vi "Histogram Window.vi"() -> ()   [LabVIEW 2019, in "Histogram Window.lvlib"]
uses:
  Histogram Window.lvlib
  Histogram Window Q Element v2.ctl
  Histogram Window Q Action v2.ctl
  Fits/Fit Plot Request Information.ctl
  <vilib>/Utility/miscctls.llb/LVPointDoubleTypeDef.ctl
  Fits/Fit Models.ctl
  <vilib>/Utility/miscctls.llb/LVPoint32TypeDef.ctl
  ALiX/Updated Plot Info.ctl
  Graphs/Plot Style 3.ctl
  Plot Histogram.ctl
  Graphs/XY Graph/XY Graph Add-Ons.lvlib
  Notebook/Notebook.lvlib
  Rich Text Box/Rich Text Box.lvlib
  Graphs/Plot Editor/Plot Editor.lvlib
panel:
  out "Histogram Graph TipStrip":string caption="Histogram TipStrip"
  out "Histogram Graph":cluster{"Axis":dbl[], "Histogram":dbl[]}[](graph)
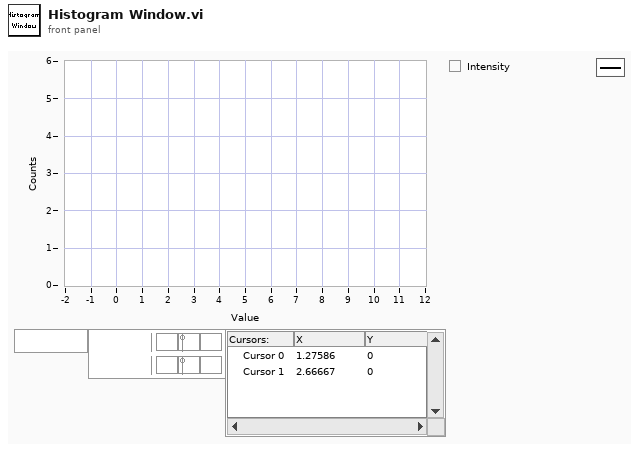
[diagram p1: front panel]
types:
  T1 = typedef "Histogram Window.lvlib/Histogram Window Q Element v2.ctl" = cluster{"Histogram Window Q Action":T2, "Data":variant}
  T2 = typedef "Histogram Window.lvlib/Histogram Window Q Action v2.ctl" = enum16{"Initialization", "Add Histogram", "Delete Histogram", "Delete Selected Histograms", "Clear Graph", "Change Bin Size", "Invert Histogram", "Update Graph", "Edit Plot", "Plot Fit", "Export XYGraph to Notebook", "Select All Plots", "Deselect All Plots", "Invert Plots Selection", "Set Style of Selected Plots", "Save Plot", "Save Selected Plots", "Save All Plots", "Quit"}
  T3 = cluster{"Event Registration Refnum":refnum<event-registration>}
  T4 = typedef "Histogram Window.lvlib/Updated Plot Info.ctl" = cluster{"Plot Index":i32, "Plot Name":string, "# Plots":i32, "Plot Style":T5}
  T5 = typedef "Plot Style 3.ctl" = cluster{"Plot Style":enum16{"unchanged", "Line", "Symbol", "Line + Symbol", "Histogram", "Histogram + Symbol"}, "Histogram Type":enum16{"unchanged", "Left Bound", "Center", "Right Bound"}, "Line Tickness":enum16{"unchanged", "Thin", "1 pixel", "2 pixel", "3 pixel", "4 pixel", "5 pixel"}, "Line Style":enum16{"unchanged", "Plain", "Long Dash", "Short Dash", "Long-Short Dash", "Long-Short-Short Dash"}, "Point Style":enum16{"unchanged", "None", "Empty Circle", "Filled Circle", "Thick Circle", "Dotted Circle", "Empty Square", "Filled Square", "Thick Square", "Dotted Square", "Small Filled Square", "Dot", "Cross", "Tiny Cross", "Large X", "Small x", "Diamond", "Small Empty Square"}, "Line Color":u32, "Point Color":u32, "Anti-aliased":bool, "Line Color Chooser":enum16{"unchanged", "Color Box", "Color List"}, "Point Color Chooser":enum16{"unchanged", "Color Box", "Color List"}, "Line Color List":string, "Point Color List":string}
  T6 = typedef "Histogram Window.lvlib/Plot Histogram.ctl" = cluster{"Plot Name":string, "Histogram":cluster{"Axis":dbl[], "Histogram":dbl[]}, "Plot Style":T5}
  T7 = typedef "LVPoint32TypeDef.ctl" = cluster{"Horizontal":i32, "Vertical":i32}
  T8 = typedef "Fit Plot Request Information.ctl" = cluster{"XY Graph Ref":refnum<vi>, "Mouse Coordinates":T9, "Fit Model":T10, "Plot Index":i32}
  T9 = typedef "LVPointDoubleTypeDef.ctl" = cluster{"X":dbl, "Y":dbl}
  T10 = typedef "Fit Models.ctl" = enum16{"Select a Fit Model...", "           Single Peak", "Gaussian", "Asymmetric Gaussian", "Lorentzian", "Asymmetric Lorentzian", "Gaussian/Lorentzian", "Lorentzian/Gaussian", "           Double Peak", "Two Gaussians", "Two Asymmetric Gaussians", "Two H-Connected Gaussians", "Two T-Connected Gaussians", "Two H-Connected Asymmetric Gaussians", "Two T-Connected Asymmetric Gaussians", "           Triple Peak", "Three Gaussians", "Three Asymmetric Gaussians", "              Decays", "1-Exponential", "IRF*PSED", "2-Exponentials", "               ACF", "2D Gaussian ACF", "2D Gaussian + Blinking ACF", "2D Gaussian + Flow ACF", "3D Gaussian ACF", "3D Gaussian + Blinking ACF", "             Multiplot", "2D Gaussian ACF & 2D Gaussian + Flow ACF"}
  T11 = cluster{"CtlRef":refnum<vi>, "Select All Plots":bool}
  T12 = typedef "XY Graph Add-Ons.lvlib/XY Graph Refnum.ctl" = refnum<vi>
  T13 = typedef "Rich Text Box.lvlib/Text Formatting.ctl" = cluster{"Font":string, "Text Color":T14, "Text Background Color":T14, "Text Style":enum16{"Regular", "Bold", "Italic", "Underline", "Strikeout"}, "Font Size (Points)":dbl, "Text Alignment":i32}
  T14 = typedef "Rich Text Box.lvlib/Text Colors.ctl" = enum16{"Unchanged", "Black", "Blue", "Gray", "Green", "Red", "White"}
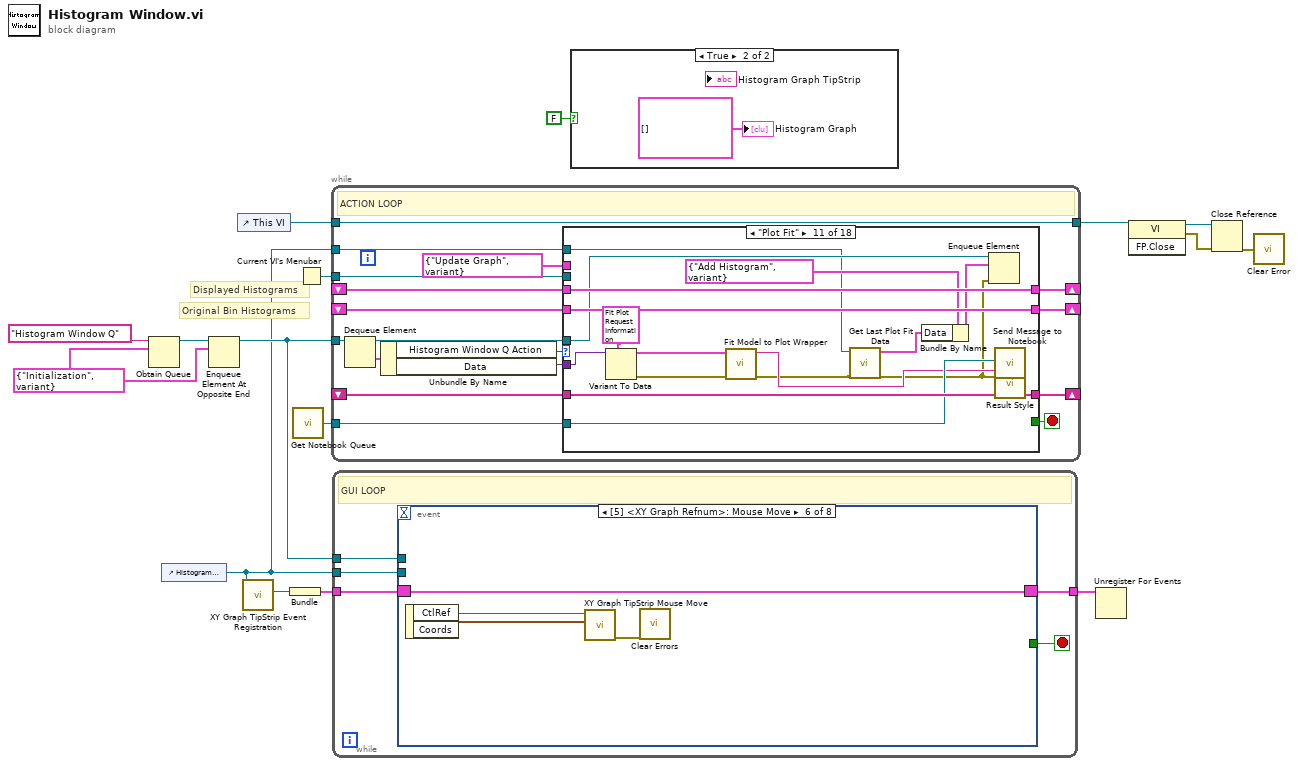
[diagram p0: block diagram]
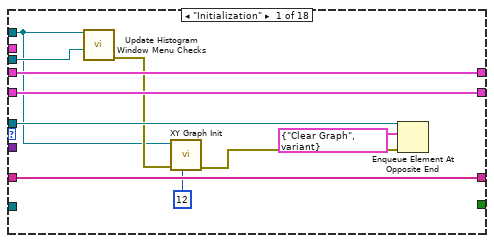
[diagram p3: hidden frame]
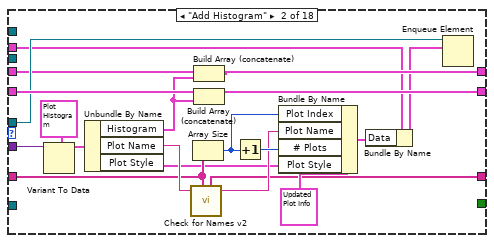
[diagram p4: hidden frame]
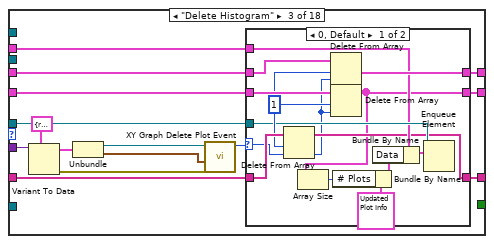
[diagram p5: hidden frame]
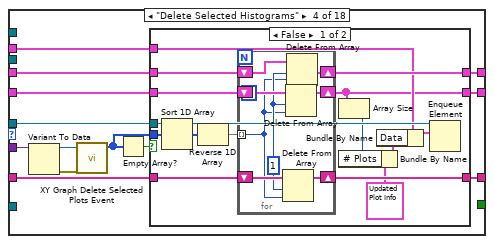
[diagram p7: hidden frame]
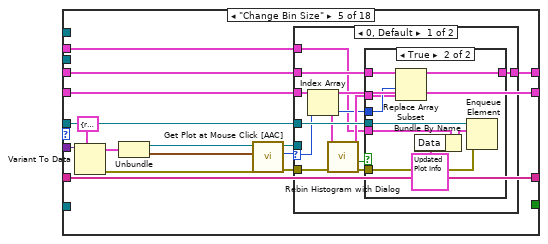
[diagram p9: hidden frame]
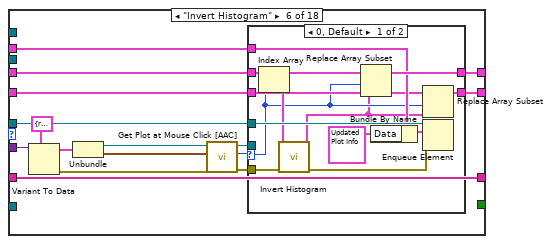
[diagram p12: hidden frame]
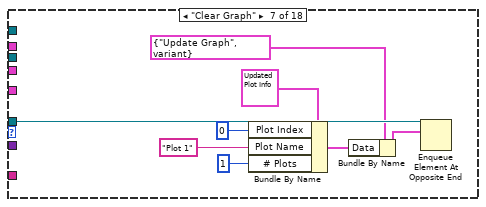
[diagram p14: hidden frame]
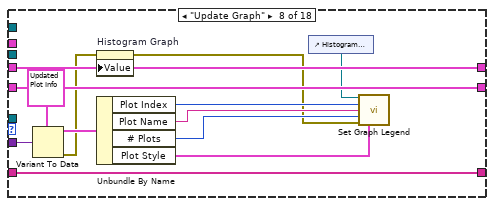
[diagram p15: hidden frame]
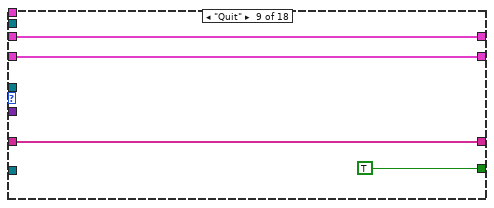
[diagram p16: hidden frame]
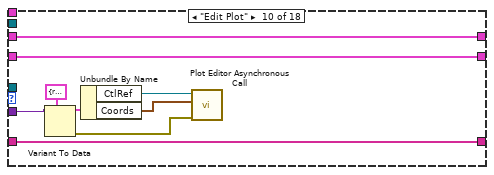
[diagram p17: hidden frame]
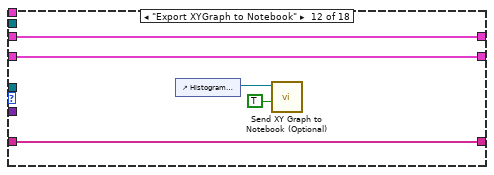
[diagram p18: hidden frame]
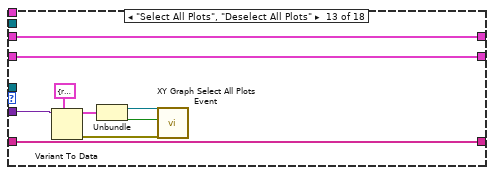
[diagram p19: hidden frame]
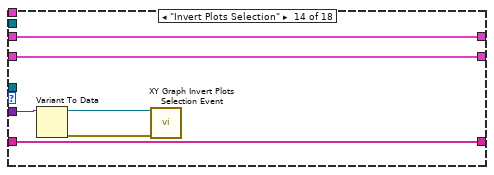
[diagram p20: hidden frame]
diagram:
  w11 = T1 {"Histogram Window Q Action"=enum."Initialization", "Data"=variant} ("ALEX TT Histogram Q Element")
  # "Displayed Histograms"
  # "Original Bin Histograms"
  n1 = Obtain Queue(name (unnamed)="Histogram Window Q", element data type=w11) -> (queue out=w15:refnum<queue>)  [unwired: 3 in, 2 out]
  n2 = control-ref of="Histogram Graph"() -> (w1:refnum<vi>)
  n3 = Enqueue Element At Opposite End(queue=w15, element=w11) -> (queue out=w12:refnum<queue>)  [unwired: 2 in, 2 out]
  n4 = control-ref of="This VI"() -> (w3:refnum<vi>)
  n5 = call "XY Graph TipStrip Event Registration.vi"("XY Graph Refnum"=w1) -> ("Event Registration Refnum"=w6:refnum<event-registration>)  [unwired: 8 in, 2 out]
  n6 = Bundle("Event Registration Refnum"=w6) -> (w9:T3)  [unwired: 1 in]
  n7 = call "Get Notebook Queue.vi"() -> ("Notebook Queue"=w10:refnum<queue>)  [unwired: 9 in]
  n8 = Current VI's Menubar() -> (w2:refnum<k9>)
  n9 = while {
    tunnel: w12 -> [w33]
    shift-right: [w27] -> _
    shift-left: _ -> [w28]
    shift-right: [w25] -> _
    shift-left: _ -> [w26]
    shift-right: [w22] -> _
    shift-left: _ -> [w23]
    tunnel: w10 -> [w20]
    tunnel: w3 -> [w19]
    tunnel: [w19] -> w7
    tunnel: w2 -> [w18]
    tunnel: w1 -> [w17]
    stop <- w30 stop-if-true
    # "ACTION LOOP"
    n10 = Dequeue Element(queue=w33) -> (queue out=w24:refnum<queue>, element=w32:T1)  [unwired: 2 in, 2 out]
    n11 = Unbundle By Name(w32) -> ("Histogram Window Q Action"=w31:T2, "Data"=w29:variant)
    n12 = case shown="\"Plot Fit\"" w31 {
      tunnel: [_ _ _ _ _ _ _ _ TRUE _ _ _ _ _ _ _ _ _] -> w30
      tunnel: w29 -> [_ w62 w78 w108 w149 w187 _ w220 _ w228 w253 _ w261 w270 w277 w296 w308 w319]
      tunnel: w28 -> [w40 w45 w71 w105 w144 w182 _ w223 w224 w236 w246 w256 w267 w273 w274 w303 w314 w325]
      tunnel: [w40 w46 w70 w104 w144 w182 _ w223 w224 w236 w246 w256 w267 w273 w274 w303 w314 w325] -> w27
      tunnel: w26 -> [w41 w63 w73 w107 w138 w173 _ w222 w225 w235 w251 w257 w266 w272 w282 w302 w313 w324]
      tunnel: [w41 w59 w72 w106 w138 w172 _ w222 w225 w235 w251 w257 w266 w272 w282 w302 w313 w324] -> w25
      tunnel: w24 -> [w43 w57 w68 w103 w139 w177 w210 _ _ _ w250 _ _ _ _ _ _ _]
      tunnel: w23 -> [w42 w56 w67 w102 w137 w176 _ w221 w226 w234 w252 w258 w265 w271 w281 w301 w312 w323]
      tunnel: [w42 w54 w66 w101 w136 w175 _ w221 w226 w234 w252 w258 w265 w271 w281 w301 w312 w323] -> w22
      tunnel: T1 {"Histogram Window Q Action"=enum."Update Graph", "Data"=variant} ("ALEX TT Histogram Q Element") -> [_ w50 w65 w100 w135 w174 _ _ _ _ _ _ _ _ _ _ _ _]
      tunnel: w20 -> [_ _ _ _ _ _ _ _ _ _ w244 _ _ _ _ w294 w306 w317]
      tunnel: w18 -> [w35 _ _ _ _ _ _ _ _ _ _ _ _ _ _ _ _ _]
      tunnel: w17 -> [w34 _ _ _ _ _ _ _ _ _ w239 _ _ _ _ _ _ _]
      frame "Initialization" {
        n13 = call "Update Histogram Window Menu Checks.vi"("menu reference"=w35, "XYGraph in"=w34) -> ("Error Out"=w36:errorcluster)  [unwired: 9 in]
        n14 = call "XY Graph Init.vi"("Max Legend Size (8)"=12 ("32bit integer"), "Error In"=w36, "XYGraph in"=w34) -> ("Error Out"=w38:errorcluster)  [unwired: 8 in]
        n15 = Enqueue Element At Opposite End(queue=w43, element=T1 {"Histogram Window Q Action"=enum."Clear Graph", "Data"=variant}, error in (no error)=w38) -> ()  [unwired: 1 in, 3 out]
      }
      frame "Add Histogram" {
        n16 = Variant To Data(type=T6 {"Plot Name"="", "Histogram"={"Axis"=[], "Histogram"=[]}, "Plot Style"={"Plot Style"=enum."Histogram + Symbol", "Histogram Type"=enum."Right Bound", "Line Tickness"=enum."unchanged", "Line Style"=enum."unchanged", "Point Style"=enum."unchanged", "Line Color"=0, "Point Color"=0, "Anti-aliased"=FALSE, "Line Color Chooser"=enum."unchanged", "Point Color Chooser"=enum."unchanged", "Line Color List"="", "Point Color List"=""}} ("output cluster"), Variant=w62) -> (data=w60:T6)  [unwired: 1 in, 1 out]
        n17 = Unbundle By Name(w60) -> ("Histogram"=w55:cluster{"Axis":dbl[], "Histogram":dbl[]}, "Plot Name"=w48:string, "Plot Style"=w44:T5)
        n18 = call "Check for Names v2.vi"("New Name"=w48, "Name List"=w45) -> ("New Name List"=w46:string[], "New Name"=w47:string)  [unwired: 4 in, 2 out]
        n19 = Array Size(array=w45) -> (size(s)=w53:i32)
        n20 = Build Array (concatenate)(w56, w55) -> (w54:cluster{"Axis":dbl[], "Histogram":dbl[]}[])
        n21 = Build Array (concatenate)(w63, w55) -> (w59:cluster{"Axis":dbl[], "Histogram":dbl[]}[])
        n22 = Increment(x=w53) -> (x+1=w58:i32)
        n23 = Bundle By Name(cluster=T4 {"Plot Index"=0, "Plot Name"="", "# Plots"=0, "Plot Style"={"Plot Style"=enum."Line + Symbol", "Histogram Type"=enum."Right Bound", "Line Tickness"=enum."Thin", "Line Style"=enum."unchanged", "Point Style"=enum."unchanged", "Line Color"=0, "Point Color"=0, "Anti-aliased"=FALSE, "Line Color Chooser"=enum."unchanged", "Point Color Chooser"=enum."unchanged", "Line Color List"="", "Point Color List"=""}} ("output cluster"), "Plot Index"=w53, "Plot Name"=w47, "# Plots"=w58, "Plot Style"=w44) -> (w51:T4)
        n24 = Bundle By Name(cluster=w50, "Data"=w51) -> (w52:T1)
        n25 = Enqueue Element(queue=w57, element=w52) -> ()  [unwired: 2 in, 3 out]
      }
      frame "Delete Histogram" {
        n26 = Variant To Data(type=cluster{"CtlRef":refnum<vi>, "Coords":T7} {"CtlRef"=refnum, "Coords"={"Horizontal"=0, "Vertical"=0}} ("output cluster"), Variant=w78) -> (data=w77:cluster{"CtlRef":refnum<vi>, "Coords":T7}, error out=w69:errorcluster)  [unwired: 1 in]
        n27 = Unbundle(w77) -> ("CtlRef"=w75:refnum<vi>, "Coords"=w74:T7)
        n28 = call "XY Graph Delete Plot Event.vi"("Error In"=w69, "Mouse Click Coordinates"=w74, "XYGraph Ref"=w75) -> ("Deleted Plot Index"=w64:i32)  [unwired: 4 in, 4 out]
        n29 = case shown="0, Default" w64 {
          selector: w64 -> [w81 _]
          tunnel: w73 -> [w92 w95]
          tunnel: [w79 w95] -> w72
          tunnel: w71 -> [w91 w94]
          tunnel: [w84 w94] -> w70
          tunnel: w68 -> [w87 _]
          tunnel: w67 -> [w90 w93]
          tunnel: [w89 w93] -> w66
          tunnel: w65 -> [w85 _]
          frame 0, Default {
            w88 = 1 ("length")
            n30 = Delete From Array(array=w91, length=w88, index=w81) -> (array with subset deleted=w84:string[])  [unwired: 1 out]
            n31 = Delete From Array(array=w90, length=w88, index=w81) -> (array with subset deleted=w89:cluster{"Axis":dbl[], "Histogram":dbl[]}[])  [unwired: 1 out]
            n32 = Delete From Array(array=w92, length=w88, index=w81) -> (array with subset deleted=w79:cluster{"Axis":dbl[], "Histogram":dbl[]}[])  [unwired: 1 out]
            n33 = Array Size(array=w79) -> (size(s)=w80:i32)
            n34 = Bundle By Name(cluster=T4 {"Plot Index"=-1, "Plot Name"="", "# Plots"=0, "Plot Style"={"Plot Style"=enum."Histogram + Symbol", "Histogram Type"=enum."Right Bound", "Line Tickness"=enum."unchanged", "Line Style"=enum."unchanged", "Point Style"=enum."unchanged", "Line Color"=0, "Point Color"=0, "Anti-aliased"=FALSE, "Line Color Chooser"=enum."unchanged", "Point Color Chooser"=enum."unchanged", "Line Color List"="", "Point Color List"=""}} ("output cluster"), "# Plots"=w80) -> (w83:T4)
            n35 = Bundle By Name(cluster=w85, "Data"=w83) -> (w86:T1)
            n36 = Enqueue Element(queue=w87, element=w86) -> ()  [unwired: 2 in, 3 out]
          }
          frame -1 {
          }
        }
      }
      frame "Delete Selected Histograms" {
        n37 = Variant To Data(Variant=w108) -> (data=w98:T12, error out=w99:errorcluster)  [unwired: 2 in]
        n38 = call "XY Graph Delete Selected Plots Event.vi"("Error In"=w99, "XYGraph Ref"=w98) -> ("Deleted Plot Indices"=w96:i32[])  [unwired: 5 in, 4 out]
        n39 = Empty Array?(array=w96) -> (empty?=w97:bool)
        n40 = case shown="False" w97 {
          tunnel: w107 -> [w123 w134]
          tunnel: [w112 w134] -> w106
          tunnel: w105 -> [w122 w133]
          tunnel: [w116 w133] -> w104
          tunnel: w103 -> [w119 _]
          tunnel: w102 -> [w121 w132]
          tunnel: [w120 w132] -> w101
          tunnel: w100 -> [w117 _]
          tunnel: w96 -> [w111 _]
          frame False {
            n41 = Sort 1D Array(array=w111) -> (sorted array=w110:i32[])
            n42 = Reverse 1D Array(array=w110) -> (reversed array=w109:i32[])
            n43 = for {
              shift-right: [w128] -> w120
              shift-left: w121 -> [w129]
              shift-right: [w125] -> w112
              shift-left: w123 -> [w131]
              shift-right: [w126] -> w116
              shift-left: w122 -> [w130]
              tunnel: w109 -> [w124] mode=indexing
              w127 = 1 ("length")
              n44 = Delete From Array(array=w130, length=w127, index=w124) -> (array with subset deleted=w126:string[])  [unwired: 1 out]
              n45 = Delete From Array(array=w131, length=w127, index=w124) -> (array with subset deleted=w125:cluster{"Axis":dbl[], "Histogram":dbl[]}[])  [unwired: 1 out]
              n46 = Delete From Array(array=w129, length=w127, index=w124) -> (array with subset deleted=w128:cluster{"Axis":dbl[], "Histogram":dbl[]}[])  [unwired: 1 out]
            }
            n47 = Array Size(array=w112) -> (size(s)=w113:i32)
            n48 = Bundle By Name(cluster=T4 {"Plot Index"=-1, "Plot Name"="", "# Plots"=0, "Plot Style"={"Plot Style"=enum."Histogram + Symbol", "Histogram Type"=enum."Right Bound", "Line Tickness"=enum."unchanged", "Line Style"=enum."unchanged", "Point Style"=enum."unchanged", "Line Color"=0, "Point Color"=0, "Anti-aliased"=FALSE, "Line Color Chooser"=enum."unchanged", "Point Color Chooser"=enum."unchanged", "Line Color List"="", "Point Color List"=""}} ("output cluster"), "# Plots"=w113) -> (w115:T4)
            n49 = Bundle By Name(cluster=w117, "Data"=w115) -> (w118:T1)
            n50 = Enqueue Element(queue=w119, element=w118) -> ()  [unwired: 2 in, 3 out]
          }
          frame True {
          }
        }
      }
      frame "Change Bin Size" {
        n51 = Variant To Data(type=cluster{"CtlRef":refnum<vi>, "Coords":T7} {"CtlRef"=refnum, "Coords"={"Horizontal"=0, "Vertical"=0}} ("output cluster"), Variant=w149) -> (data=w148:cluster{"CtlRef":refnum<vi>, "Coords":T7}, error out=w143:errorcluster)  [unwired: 1 in]
        n52 = Unbundle(w148) -> ("CtlRef"=w146:refnum<vi>, "Coords"=w145:T7)
        n53 = call "Get Plot at Mouse Click [AAC].vi"("error in (no error)"=w143, "Mouse Click Coordinates"=w145, "XYGraph Ref"=w146) -> ("error out"=w141:errorcluster, "Plot at Coordinates"=w142:i32, "XYGraph Ref"=w140:T12)  [unwired: 2 in, 4 out]
        n54 = case shown="0, Default" w142 {
          selector: w142 -> [w151 _]
          tunnel: w141 -> [w160 _]
          tunnel: w140 -> [_ _]
          tunnel: w139 -> [w159 _]
          tunnel: w138 -> [w157 _]
          tunnel: w137 -> [w154 w171]
          tunnel: [w153 w171] -> w136
          tunnel: w135 -> [w150 _]
          frame 0, Default {
            n55 = Index Array(array=w157, index=w151) -> (element=w156:cluster{"Axis":dbl[], "Histogram":dbl[]})
            n56 = call "Rebin Histogram with Dialog.vi"("error in (no error)"=w160, "Original Bin Histogram"=w156) -> ("error out"=w158:errorcluster, "OK?"=w155:bool, "Rebinned Histogram"=w152:cluster{"Axis":dbl[], "Histogram":dbl[]})  [unwired: 7 in]
            n57 = case shown="True" w155 {
              tunnel: w159 -> [_ w170]
              tunnel: w158 -> [_ w169]
              tunnel: w154 -> [w161 w168]
              tunnel: [w161 w167] -> w153
              tunnel: w152 -> [_ w165]
              tunnel: w151 -> [_ w166]
              tunnel: w150 -> [_ w164]
              frame False {
              }
              frame True {
                n58 = Replace Array Subset(array=w168, new element=w165, index=w166) -> (w167:cluster{"Axis":dbl[], "Histogram":dbl[]}[])
                n59 = Bundle By Name(cluster=w164, "Data"=T4 {"Plot Index"=-1, "Plot Name"="", "# Plots"=0, "Plot Style"={"Plot Style"=enum."Histogram + Symbol", "Histogram Type"=enum."Right Bound", "Line Tickness"=enum."unchanged", "Line Style"=enum."unchanged", "Point Style"=enum."unchanged", "Line Color"=0, "Point Color"=0, "Anti-aliased"=FALSE, "Line Color Chooser"=enum."unchanged", "Point Color Chooser"=enum."unchanged", "Line Color List"="", "Point Color List"=""}} ("Updated Plot Info")) -> (w163:T1)
                n60 = Enqueue Element(queue=w170, element=w163, error in (no error)=w169) -> ()  [unwired: 1 in, 3 out]
              }
            }
          }
          frame -1 {
          }
        }
      }
      frame "Invert Histogram" {
        n61 = Variant To Data(type=cluster{"CtlRef":refnum<vi>, "Coords":T7} {"CtlRef"=refnum, "Coords"={"Horizontal"=0, "Vertical"=0}} ("output cluster"), Variant=w187) -> (data=w186:cluster{"CtlRef":refnum<vi>, "Coords":T7}, error out=w181:errorcluster)  [unwired: 1 in]
        n62 = Unbundle(w186) -> ("CtlRef"=w184:refnum<vi>, "Coords"=w183:T7)
        n63 = call "Get Plot at Mouse Click [AAC].vi"("error in (no error)"=w181, "Mouse Click Coordinates"=w183, "XYGraph Ref"=w184) -> ("error out"=w179:errorcluster, "Plot at Coordinates"=w180:i32, "XYGraph Ref"=w178:T12)  [unwired: 2 in, 4 out]
        n64 = case shown="0, Default" w180 {
          selector: w180 -> [w190 _]
          tunnel: w179 -> [w200 _]
          tunnel: w178 -> [_ _]
          tunnel: w177 -> [w199 _]
          tunnel: w176 -> [w195 w202]
          tunnel: [w197 w202] -> w175
          tunnel: w174 -> [w196 _]
          tunnel: w173 -> [w191 w201]
          tunnel: [w188 w201] -> w172
          frame 0, Default {
            n65 = Index Array(array=w195, index=w190) -> (element=w194:cluster{"Axis":dbl[], "Histogram":dbl[]})
            n66 = call "Invert Histogram.vi"("error in (no error)"=w200, "Histogram"=w194) -> ("error out"=w198:errorcluster, "Inverted Histogram"=w189:cluster{"Axis":dbl[], "Histogram":dbl[]})  [unwired: 8 in]
            n67 = Replace Array Subset(array=w195, new element=w189, index=w190) -> (w197:cluster{"Axis":dbl[], "Histogram":dbl[]}[])
            n68 = Bundle By Name(cluster=w196, "Data"=T4 {"Plot Index"=-1, "Plot Name"="", "# Plots"=0, "Plot Style"={"Plot Style"=enum."Histogram + Symbol", "Histogram Type"=enum."Right Bound", "Line Tickness"=enum."unchanged", "Line Style"=enum."unchanged", "Point Style"=enum."unchanged", "Line Color"=0, "Point Color"=0, "Anti-aliased"=FALSE, "Line Color Chooser"=enum."unchanged", "Point Color Chooser"=enum."unchanged", "Line Color List"="", "Point Color List"=""}} ("output cluster")) -> (w193:T1)
            n69 = Replace Array Subset(array=w191, new element=w189, index=w190) -> (w188:cluster{"Axis":dbl[], "Histogram":dbl[]}[])
            n70 = Enqueue Element(queue=w199, element=w193, error in (no error)=w198) -> ()  [unwired: 1 in, 3 out]
          }
          frame -1 {
          }
        }
      }
      frame "Clear Graph" {
        n71 = Bundle By Name(cluster=T4 {"Plot Index"=0, "Plot Name"="", "# Plots"=0, "Plot Style"={"Plot Style"=enum."Histogram + Symbol", "Histogram Type"=enum."Right Bound", "Line Tickness"=enum."unchanged", "Line Style"=enum."unchanged", "Point Style"=enum."unchanged", "Line Color"=0, "Point Color"=0, "Anti-aliased"=FALSE, "Line Color Chooser"=enum."unchanged", "Point Color Chooser"=enum."unchanged", "Line Color List"="", "Point Color List"=""}} ("output cluster"), "Plot Index"=0, "Plot Name"="Plot 1", "# Plots"=1 ("# Legend Rows")) -> (w206:T4)
        n72 = Bundle By Name(cluster=T1 {"Histogram Window Q Action"=enum."Update Graph", "Data"=variant} ("ALEX TT Histogram Q Element"), "Data"=w206) -> (w208:T1)
        n73 = Enqueue Element At Opposite End(queue=w210, element=w208) -> ()  [unwired: 2 in, 3 out]
      }
      frame "Update Graph" {
        n74 = Variant To Data(type=T4 {"Plot Index"=0, "Plot Name"="", "# Plots"=0, "Plot Style"={"Plot Style"=enum."Histogram + Symbol", "Histogram Type"=enum."Right Bound", "Line Tickness"=enum."unchanged", "Line Style"=enum."unchanged", "Point Style"=enum."unchanged", "Line Color"=0, "Point Color"=0, "Anti-aliased"=FALSE, "Line Color Chooser"=enum."unchanged", "Point Color Chooser"=enum."unchanged", "Line Color List"="", "Point Color List"=""}} ("output cluster"), Variant=w220) -> (data=w218:T4, error out=w213:errorcluster)  [unwired: 1 in]
        n75 = property on="Histogram Graph" class="XYGraph (strict)"(error in=w213, "Value"=w221) -> (error out=w212:errorcluster)  [unwired: 1 in, 1 out]
        n76 = Unbundle By Name(w218) -> ("Plot Index"=w217:i32, "Plot Name"=w215:string, "# Plots"=w216:i32, "Plot Style"=w211:T5)
        n77 = control-ref of="Histogram Graph"() -> (w214:refnum<vi>)
        n78 = call "Set Graph Legend.vi"("XYGraph in"=w214, "Active Plot"=w217, "Plot Name"=w215, "# Plots"=w216, "error in (no error)"=w212, "Plot Style"=w211) -> ()  [unwired: 9 in, 1 out]
      }
      frame "Quit" {
      }
      frame "Edit Plot" {
        n79 = Variant To Data(type=cluster{"CtlRef":refnum<vi>, "Coords":T7} {"CtlRef"=refnum, "Coords"={"Horizontal"=0, "Vertical"=0}} ("output cluster"), Variant=w228) -> (data=w230:cluster{"CtlRef":refnum<vi>, "Coords":T7}, error out=w232:errorcluster)  [unwired: 1 in]
        n80 = Unbundle By Name(w230) -> ("CtlRef"=w233:refnum<vi>, "Coords"=w231:T7)
        n81 = call "Plot Editor Asynchronous Call.vi"("error in (no error)"=w232, "Coords"=w231, "XYGraph in"=w233) -> ()  [unwired: 5 in, 4 out]
      }
      frame "Plot Fit" {
        n82 = Variant To Data(type=T8 {"XY Graph Ref"=refnum, "Mouse Coordinates"={"X"=0.0, "Y"=0.0}, "Fit Model"=enum."Select a Fit Model...", "Plot Index"=-1} ("output cluster"), Variant=w253) -> (data=w242:T8, error out=w240:errorcluster)  [unwired: 1 in]
        n83 = call "Fit Model to Plot Wrapper.vi"("error in (no error)"=w240, "Fit Plot Info"=w242) -> ("error out"=w238:errorcluster, "Fit Result String"=w243:string)  [unwired: 8 in]
        n84 = call "Get Last Plot Fit Data.vi"("error in (no error)"=w238, "XYGraph in"=w239) -> ("error out"=w237:errorcluster, "Last Fit Data"=w247:T6)  [unwired: 8 in]
        n85 = Bundle By Name(cluster=T1 {"Histogram Window Q Action"=enum."Add Histogram", "Data"=variant} ("element"), "Data"=w247) -> (w248:T1)
        n86 = Enqueue Element(queue=w250, element=w248, error in (no error)=w237) -> ()  [unwired: 1 in, 3 out]
        n87 = call "Result Style.vi"() -> ("Default Text Formatting"=w241:T13)
        n88 = call "Send Message to Notebook.vi"("Notebook Queue"=w244, "Message"=w243, "Error In"=w237, "Text Formatting"=w241) -> ()  [unwired: 15 in, 1 out]
      }
      frame "Export XYGraph to Notebook" {
        n89 = control-ref of="Histogram Graph"() -> (w255:refnum<vi>)
        n90 = call "Send XY Graph to Notebook (Optional).vi"("Send Graph to Notebook?"=TRUE, "XYGraph in"=w255) -> ()  [unwired: 9 in, 1 out]
      }
      frame "Select All Plots", "Deselect All Plots" {
        n91 = Variant To Data(type=T11 {"CtlRef"=refnum, "Select All Plots"=TRUE} ("output cluster"), Variant=w261) -> (data=w264:T11, error out=w259:errorcluster)  [unwired: 1 in]
        n92 = Unbundle(w264) -> ("CtlRef"=w263:refnum<vi>, "Select All Plots"=w262:bool)
        n93 = call "XY Graph Select All Plots Event.vi"("Error In"=w259, "Select (T)/Deselect"=w262, "XYGraph Ref"=w263) -> ()  [unwired: 5 in, 4 out]
      }
      frame "Invert Plots Selection" {
        n94 = Variant To Data(Variant=w270) -> (data=w269:T12, error out=w268:errorcluster)  [unwired: 2 in]
        n95 = call "XY Graph Invert Plots Selection Event.vi"("Error In"=w268, "XYGraph Ref"=w269) -> ()  [unwired: 6 in, 4 out]
      }
      frame "Set Style of Selected Plots" {
        n96 = Variant To Data(type=refnum<vi> refnum ("XYGraph Ref"), Variant=w277) -> (data=w275:refnum<vi>)  [unwired: 1 in, 1 out]
        n97 = call "Plot Style Chooser Dialog.vi"() -> ("Plot Style out"=w280:T5, "Cancelled?"=w279:bool, "Error Out"=w278:errorcluster)  [unwired: 7 in]
        n98 = case shown="True" w279 {
          tunnel: w275 -> [_ w285]
          tunnel: w280 -> [_ w284]
          tunnel: w278 -> [_ w283]
          frame False {
          }
          frame True {
            n99 = call "XY Graph Set Style of Selected Plots.vi"("Error In"=w283, "Plot Style"=w284, "XYGraph Ref"=w285) -> ()  [unwired: 5 in, 4 out]
          }
        }
      }
      frame "Save Plot" {
        n100 = Variant To Data(type=cluster{"CtlRef":refnum<vi>, "Coords":T7} {"CtlRef"=refnum, "Coords"={"Horizontal"=0, "Vertical"=0}} ("output cluster"), Variant=w296) -> (data=w299:cluster{"CtlRef":refnum<vi>, "Coords":T7}, error out=w295:errorcluster)  [unwired: 1 in]
        n101 = Unbundle By Name(w299) -> ("CtlRef"=w297:refnum<vi>, "Coords"=w298:T7)
        n102 = call "XY Graph Save Plot Event.vi"("Error In"=w295, "Mouse Click Coordinates"=w298, "XYGraph Ref"=w297) -> ("Error Out"=w289:errorcluster, "Message"=w292:string, "File Path"=w286:path, "Plot Name"=w287:string)  [unwired: 3 in, 2 out]
        n103 = Format Into String(format string=" from %s saved as %s", initial string=w292, error in=w289, w287, w286) -> (resulting string=w290:string, error out=w288:errorcluster)
        n104 = call "Message Style.vi"() -> ("Message Formatting"=w293:T13)
        n105 = call "Send Message to Notebook.vi"("Notebook Queue"=w294, "Message"=w290, "Error In"=w288, "Text Formatting"=w293) -> ()  [unwired: 15 in, 1 out]
      }
      frame "Save Selected Plots" {
        n106 = Variant To Data(Variant=w308) -> (data=w311:T12, error out=w309:errorcluster)  [unwired: 2 in]
        n107 = call "XY Graph Save Selected Plots Event.vi"("Error In"=w309, "Save All Plots? (T)"=FALSE, "XYGraph Ref"=w311) -> ("Error Out"=w305:errorcluster, "Message"=w304:string)  [unwired: 3 in, 4 out]
        n108 = call "Message Style.vi"() -> ("Message Formatting"=w307:T13)
        n109 = call "Send Message to Notebook.vi"("Notebook Queue"=w306, "Message"=w304, "Error In"=w305, "Text Formatting"=w307) -> ()  [unwired: 15 in, 1 out]
      }
      frame "Save All Plots" {
        n110 = Variant To Data(Variant=w319) -> (data=w322:T12, error out=w320:errorcluster)  [unwired: 2 in]
        n111 = call "XY Graph Save Selected Plots Event.vi"("Error In"=w320, "Save All Plots? (T)"=TRUE, "XYGraph Ref"=w322) -> ("Error Out"=w316:errorcluster, "Message"=w315:string)  [unwired: 3 in, 4 out]
        n112 = call "Message Style.vi"() -> ("Message Formatting"=w318:T13)
        n113 = call "Send Message to Notebook.vi"("Notebook Queue"=w317, "Message"=w315, "Error In"=w316, "Text Formatting"=w318) -> ()  [unwired: 15 in, 1 out]
      }
    }
  }
  n114 = while {
    tunnel: w12 -> [w329]
    tunnel: w9 -> [w327]
    tunnel: [w328] -> w5
    tunnel: w1 -> [w326]
    stop <- w330 stop-if-true
    # "GUI LOOP"
    n115 = event shown="[5] <XY Graph Refnum>: Mouse Move" {
      selector: w327 -> [_ _ _ w552 w557 w559 _ _]
      dyn-events: [_ _ _ w551 w556 w559 _ _] -> w328
      timeout: _ -> [_ _ _ _ _ _ _ _]
      tunnel: [_ _ _ _ _ _ w563 w613] -> w330
      tunnel: w329 -> [_ w338 w547 _ _ _ w565 w612]
      tunnel: w326 -> [_ _ _ _ _ _ w564 _]
      event "Histogram Graph": Shortcut Menu Activation? {
        n116 = event-data() -> ("CtlRef"=w331:refnum<vi>, "MenuRef"=w333:refnum<k9>)  [unwired: 1 in]
        n117 = call "Use Custom Object Menu.vi"("Menu in"=w333, "CtlRef"=w331) -> ("error out"=w334:errorcluster, "Menu out"=w332:refnum<k9>)  [unwired: 7 in, 1 out]
        n118 = call "XY Graph Check-Uncheck Menu Items.vi"("Error In"=w334, "Menu in"=w332, "XY Graph Refnum"=w331) -> ()  [unwired: 7 in, 2 out]
        n119 = event-data("Discard?"=FALSE) -> ()  [unwired: 1 in, 1 out]
      }
      event "Histogram Graph": Shortcut Menu Selection (User) {
        n120 = event-data() -> ("CtlRef"=w341:refnum<vi>, "ItemTag"=w340:string, "Coords"=w339:T7)  [unwired: 1 in]
        n121 = case shown="\"\", Default" w340 {
          tunnel: w341 -> [_ w344 _ _ w353 w355 w363 w369 w375 w377 w385 w387 w395 w397 w401 w405 _ w415 w423 w431 w439 w447 w455 w463 w471 w479 w487 w495 w503 w511 w519 w527 w535 _ _ w539 w540]
          tunnel: w339 -> [_ w343 _ _ w352 _ w362 w368 w374 _ _ _ _ _ _ _ _ w414 w422 w430 w438 w446 w454 w462 w470 w478 w486 w494 w502 w510 w518 w526 w534 _ _ _ _]
          tunnel: w338 -> [_ w348 _ _ w354 w358 w364 w370 w376 w380 w386 w390 w396 w400 w404 w408 _ w416 w424 w432 w440 w448 w456 w464 w472 w480 w488 w496 w504 w512 w520 w528 w536 w538 _ _ _]
          tunnel: T1 {"Histogram Window Q Action"=enum."Plot Fit", "Data"=variant} ("ALEX TT Histogram Q Element") -> [_ _ _ _ _ _ _ _ _ _ _ _ _ _ _ _ _ w411 w418 w426 w434 w442 w450 w458 w466 w474 w482 w490 w498 w506 w514 w522 w531 _ _ _ _]
          tunnel: T8 {"XY Graph Ref"=refnum, "Mouse Coordinates"={"X"=0.0, "Y"=0.0}, "Fit Model"=enum."Select a Fit Model...", "Plot Index"=-1} ("output cluster") -> [_ _ _ _ _ _ _ _ _ _ _ _ _ _ _ _ _ w409 w417 w425 w433 w441 w449 w457 w465 w473 w481 w489 w497 w505 w513 w521 w530 _ _ _ _]
          frame "", Default {
          }
          frame "Edit Plot" {
            n122 = Bundle By Name(cluster=cluster{"CtlRef":refnum<vi>, "Coords":T7} {"CtlRef"=refnum, "Coords"={"Horizontal"=0, "Vertical"=0}} ("output cluster"), "CtlRef"=w344, "Coords"=w343) -> (w346:cluster{"CtlRef":refnum<vi>, "Coords":T7})
            n123 = Bundle By Name(cluster=T1 {"Histogram Window Q Action"=enum."Edit Plot", "Data"=variant} ("ALEX TT Histogram Q Element"), "Data"=w346) -> (w342:T1)
            n124 = Enqueue Element(queue=w348, element=w342) -> ()  [unwired: 2 in, 3 out]
          }
          frame "Send Plot to Advanced Plot Window" {
          }
          frame "Send Graph to Advanced Plot Window" {
          }
          frame "Delete Plot" {
            n125 = Bundle("CtlRef"=w353, "Coords"=w352) -> (w350:cluster{"CtlRef":refnum<vi>, "Coords":T7})  [unwired: 1 in]
            n126 = Bundle By Name(cluster=T1 {"Histogram Window Q Action"=enum."Delete Histogram", "Data"=variant} ("ALEX TT Histogram Q Element"), "Data"=w350) -> (w351:T1)
            n127 = Enqueue Element(queue=w354, element=w351) -> ()  [unwired: 2 in, 3 out]
          }
          frame "Delete Selected Plots" {
            n128 = Bundle By Name(cluster=T1 {"Histogram Window Q Action"=enum."Delete Selected Histograms", "Data"=variant} ("ALEX TT Histogram Q Element"), "Data"=w355) -> (w357:T1)
            n129 = Enqueue Element(queue=w358, element=w357) -> ()  [unwired: 2 in, 3 out]
          }
          frame "Save Plot" {
            n130 = Bundle("CtlRef"=w363, "Coords"=w362) -> (w360:cluster{"CtlRef":refnum<vi>, "Coords":T7})  [unwired: 1 in]
            n131 = Bundle By Name(cluster=T1 {"Histogram Window Q Action"=enum."Save Plot", "Data"=variant} ("ALEX TT Histogram Q Element"), "Data"=w360) -> (w361:T1)
            n132 = Enqueue Element(queue=w364, element=w361) -> ()  [unwired: 2 in, 3 out]
          }
          frame "Rebin Histogram" {
            n133 = Bundle("CtlRef"=w369, "Coords"=w368) -> (w366:cluster{"CtlRef":refnum<vi>, "Coords":T7})  [unwired: 1 in]
            n134 = Bundle By Name(cluster=T1 {"Histogram Window Q Action"=enum."Change Bin Size", "Data"=variant} ("ALEX TT Histogram Q Element"), "Data"=w366) -> (w367:T1)
            n135 = Enqueue Element(queue=w370, element=w367) -> ()  [unwired: 2 in, 3 out]
          }
          frame "Invert Histogram" {
            n136 = Bundle("CtlRef"=w375, "Coords"=w374) -> (w372:cluster{"CtlRef":refnum<vi>, "Coords":T7})  [unwired: 1 in]
            n137 = Bundle By Name(cluster=T1 {"Histogram Window Q Action"=enum."Invert Histogram", "Data"=variant} ("ALEX TT Histogram Q Element"), "Data"=w372) -> (w373:T1)
            n138 = Enqueue Element(queue=w376, element=w373) -> ()  [unwired: 2 in, 3 out]
          }
          frame "Clear Graph" {
            n139 = Bundle By Name(cluster=T1 {"Histogram Window Q Action"=enum."Clear Graph", "Data"=variant} ("ALEX TT Histogram Q Element"), "Data"=w377) -> (w379:T1)
            n140 = Enqueue Element(queue=w380, element=w379) -> ()  [unwired: 2 in, 3 out]
          }
          frame "Select All Plots" {
            n141 = Bundle("CtlRef"=w385, TRUE) -> (w383:cluster{"CtlRef":refnum<vi>, bool})  [unwired: 1 in]
            n142 = Bundle By Name(cluster=T1 {"Histogram Window Q Action"=enum."Select All Plots", "Data"=variant} ("ALEX TT Histogram Q Element"), "Data"=w383) -> (w384:T1)
            n143 = Enqueue Element(queue=w386, element=w384) -> ()  [unwired: 2 in, 3 out]
          }
          frame "Invert Plots Selection" {
            n144 = Bundle By Name(cluster=T1 {"Histogram Window Q Action"=enum."Invert Plots Selection", "Data"=variant} ("element"), "Data"=w387) -> (w388:T1)
            n145 = Enqueue Element(queue=w390, element=w388) -> ()  [unwired: 2 in, 3 out]
          }
          frame "Deselect All Plots" {
            n146 = Bundle("CtlRef"=w395, FALSE) -> (w393:cluster{"CtlRef":refnum<vi>, bool})  [unwired: 1 in]
            n147 = Bundle By Name(cluster=T1 {"Histogram Window Q Action"=enum."Select All Plots", "Data"=variant} ("ALEX TT Histogram Q Element"), "Data"=w393) -> (w394:T1)
            n148 = Enqueue Element(queue=w396, element=w394) -> ()  [unwired: 2 in, 3 out]
          }
          frame "Set Style of Selected Plots" {
            n149 = Bundle By Name(cluster=T1 {"Histogram Window Q Action"=enum."Set Style of Selected Plots", "Data"=variant} ("ALEX TT Histogram Q Element"), "Data"=w397) -> (w399:T1)
            n150 = Enqueue Element(queue=w400, element=w399) -> ()  [unwired: 2 in, 3 out]
          }
          frame "Save Selected Plots" {
            n151 = Bundle By Name(cluster=T1 {"Histogram Window Q Action"=enum."Save Selected Plots", "Data"=variant} ("ALEX TT Histogram Q Element"), "Data"=w401) -> (w403:T1)
            n152 = Enqueue Element(queue=w404, element=w403) -> ()  [unwired: 2 in, 3 out]
          }
          frame "Save All Plots" {
            n153 = Bundle By Name(cluster=T1 {"Histogram Window Q Action"=enum."Save All Plots", "Data"=variant} ("ALEX TT Histogram Q Element"), "Data"=w405) -> (w407:T1)
            n154 = Enqueue Element(queue=w408, element=w407) -> ()  [unwired: 2 in, 3 out]
          }
          frame "----------- Fits -----------" {
          }
          frame "Gaussian" {
            n155 = Bundle By Name(cluster=w409, "XY Graph Ref"=w415, "Mouse Coordinates"=w414, "Fit Model"=Fit_Models."Gaussian") -> (w413:T8)
            n156 = Bundle By Name(cluster=w411, "Data"=w413) -> (w410:T1)
            n157 = Enqueue Element(queue=w416, element=w410) -> ()  [unwired: 2 in, 3 out]
          }
          frame "Lorentzian" {
            n158 = Bundle By Name(cluster=w417, "XY Graph Ref"=w423, "Mouse Coordinates"=w422, "Fit Model"=Fit_Models."Lorentzian") -> (w420:T8)
            n159 = Bundle By Name(cluster=w418, "Data"=w420) -> (w421:T1)
            n160 = Enqueue Element(queue=w424, element=w421) -> ()  [unwired: 2 in, 3 out]
          }
          frame "Asymmetric Gaussian" {
            n161 = Bundle By Name(cluster=w425, "XY Graph Ref"=w431, "Mouse Coordinates"=w430, "Fit Model"=Fit_Models."Asymmetric Gaussian") -> (w428:T8)
            n162 = Bundle By Name(cluster=w426, "Data"=w428) -> (w429:T1)
            n163 = Enqueue Element(queue=w432, element=w429) -> ()  [unwired: 2 in, 3 out]
          }
          frame "Asymmetric Lorentzian" {
            n164 = Bundle By Name(cluster=w433, "XY Graph Ref"=w439, "Mouse Coordinates"=w438, "Fit Model"=Fit_Models."Asymmetric Lorentzian") -> (w436:T8)
            n165 = Bundle By Name(cluster=w434, "Data"=w436) -> (w437:T1)
            n166 = Enqueue Element(queue=w440, element=w437) -> ()  [unwired: 2 in, 3 out]
          }
          frame "Gaussian/Lorentzian" {
            n167 = Bundle By Name(cluster=w441, "XY Graph Ref"=w447, "Mouse Coordinates"=w446, "Fit Model"=Fit_Models."Gaussian/Lorentzian") -> (w444:T8)
            n168 = Bundle By Name(cluster=w442, "Data"=w444) -> (w445:T1)
            n169 = Enqueue Element(queue=w448, element=w445) -> ()  [unwired: 2 in, 3 out]
          }
          frame "Lorentzian/Gaussian" {
            n170 = Bundle By Name(cluster=w449, "XY Graph Ref"=w455, "Mouse Coordinates"=w454, "Fit Model"=Fit_Models."Lorentzian/Gaussian") -> (w452:T8)
            n171 = Bundle By Name(cluster=w450, "Data"=w452) -> (w453:T1)
            n172 = Enqueue Element(queue=w456, element=w453) -> ()  [unwired: 2 in, 3 out]
          }
          frame "1-Exponential" {
            n173 = Bundle By Name(cluster=w457, "XY Graph Ref"=w463, "Mouse Coordinates"=w462, "Fit Model"=Fit_Models."1-Exponential") -> (w460:T8)
            n174 = Bundle By Name(cluster=w458, "Data"=w460) -> (w461:T1)
            n175 = Enqueue Element(queue=w464, element=w461) -> ()  [unwired: 2 in, 3 out]
          }
          frame "2-Exponentials" {
            n176 = Bundle By Name(cluster=w465, "XY Graph Ref"=w471, "Mouse Coordinates"=w470, "Fit Model"=Fit_Models."2-Exponentials") -> (w468:T8)
            n177 = Bundle By Name(cluster=w466, "Data"=w468) -> (w469:T1)
            n178 = Enqueue Element(queue=w472, element=w469) -> ()  [unwired: 2 in, 3 out]
          }
          frame "Two Gaussians" {
            n179 = Bundle By Name(cluster=w473, "XY Graph Ref"=w479, "Mouse Coordinates"=w478, "Fit Model"=Fit_Models."Two Gaussians") -> (w476:T8)
            n180 = Bundle By Name(cluster=w474, "Data"=w476) -> (w477:T1)
            n181 = Enqueue Element(queue=w480, element=w477) -> ()  [unwired: 2 in, 3 out]
          }
          frame "Two Asymmetric Gaussians" {
            n182 = Bundle By Name(cluster=w481, "XY Graph Ref"=w487, "Mouse Coordinates"=w486, "Fit Model"=Fit_Models."Two Asymmetric Gaussians") -> (w484:T8)
            n183 = Bundle By Name(cluster=w482, "Data"=w484) -> (w485:T1)
            n184 = Enqueue Element(queue=w488, element=w485) -> ()  [unwired: 2 in, 3 out]
          }
          frame "Two H-Connected Gaussians" {
            n185 = Bundle By Name(cluster=w489, "XY Graph Ref"=w495, "Mouse Coordinates"=w494, "Fit Model"=Fit_Models."Two H-Connected Gaussians") -> (w492:T8)
            n186 = Bundle By Name(cluster=w490, "Data"=w492) -> (w493:T1)
            n187 = Enqueue Element(queue=w496, element=w493) -> ()  [unwired: 2 in, 3 out]
          }
          frame "Two T-Connected Gaussians" {
            n188 = Bundle By Name(cluster=w497, "XY Graph Ref"=w503, "Mouse Coordinates"=w502, "Fit Model"=Fit_Models."Two T-Connected Gaussians") -> (w500:T8)
            n189 = Bundle By Name(cluster=w498, "Data"=w500) -> (w501:T1)
            n190 = Enqueue Element(queue=w504, element=w501) -> ()  [unwired: 2 in, 3 out]
          }
          frame "Two H-Connected Asymmetric Gaussians" {
            n191 = Bundle By Name(cluster=w505, "XY Graph Ref"=w511, "Mouse Coordinates"=w510, "Fit Model"=Fit_Models."Two H-Connected Asymmetric Gaussians") -> (w508:T8)
            n192 = Bundle By Name(cluster=w506, "Data"=w508) -> (w509:T1)
            n193 = Enqueue Element(queue=w512, element=w509) -> ()  [unwired: 2 in, 3 out]
          }
          frame "Two T-Connected Asymmetric Gaussians" {
            n194 = Bundle By Name(cluster=w513, "XY Graph Ref"=w519, "Mouse Coordinates"=w518, "Fit Model"=Fit_Models."Two T-Connected Asymmetric Gaussians") -> (w516:T8)
            n195 = Bundle By Name(cluster=w514, "Data"=w516) -> (w517:T1)
            n196 = Enqueue Element(queue=w520, element=w517) -> ()  [unwired: 2 in, 3 out]
          }
          frame "Three Gaussians" {
            n197 = Bundle By Name(cluster=w521, "XY Graph Ref"=w527, "Mouse Coordinates"=w526, "Fit Model"=Fit_Models."Three Gaussians") -> (w524:T8)
            n198 = Bundle By Name(cluster=w522, "Data"=w524) -> (w525:T1)
            n199 = Enqueue Element(queue=w528, element=w525) -> ()  [unwired: 2 in, 3 out]
          }
          frame "Three Asymmetric Gaussians" {
            n200 = Bundle By Name(cluster=w530, "XY Graph Ref"=w535, "Mouse Coordinates"=w534, "Fit Model"=Fit_Models."Three Asymmetric Gaussians") -> (w532:T8)
            n201 = Bundle By Name(cluster=w531, "Data"=w532) -> (w533:T1)
            n202 = Enqueue Element(queue=w536, element=w533) -> ()  [unwired: 2 in, 3 out]
          }
          frame "Export Image to Notebook" {
            n203 = Enqueue Element(queue=w538, element=T1 {"Histogram Window Q Action"=enum."Export XYGraph to Notebook", "Data"=variant}) -> ()  [unwired: 2 in, 3 out]
          }
          frame "-------------" {
          }
          frame "Grid" {
            n204 = call "XY Graph Show-Hide Grid Event.vi"("XYGraph Ref in"=w539) -> ()  [unwired: 7 in, 4 out]
          }
          frame "Tool Panels" {
            n205 = call "XY Graph Show-Hide Tool Panels Event.vi"("XYGraph in"=w540) -> ()  [unwired: 8 in, 3 out]
          }
        }
      }
      event Pane Size {
        n206 = event-data() -> ()  [unwired: 1 in, 1 out]
        n207 = control-ref of="Histogram Graph"() -> (w542:refnum<vi>)
        n208 = call "XY Graph Number of Plots.vi"("XYGraph in"=w542) -> ("# Plots"=w541:i32)  [unwired: 9 in, 1 out]
        n209 = Bundle By Name(cluster=T4 {"Plot Index"=-1, "Plot Name"="", "# Plots"=0, "Plot Style"={"Plot Style"=enum."Histogram + Symbol", "Histogram Type"=enum."Right Bound", "Line Tickness"=enum."unchanged", "Line Style"=enum."unchanged", "Point Style"=enum."unchanged", "Line Color"=0, "Point Color"=0, "Anti-aliased"=FALSE, "Line Color Chooser"=enum."unchanged", "Point Color Chooser"=enum."unchanged", "Line Color List"="", "Point Color List"=""}} ("Updated Plot Info"), "# Plots"=w541) -> (w543:T4)
        n210 = Bundle By Name(cluster=T1 {"Histogram Window Q Action"=enum."Update Graph", "Data"=variant} ("element"), "Data"=w543) -> (w545:T1)
        n211 = Enqueue Element(queue=w547, element=w545) -> ()  [unwired: 2 in, 3 out]
      }
      event Mouse Enter {
        n212 = event-data() -> ("CtlRef"=w550:refnum<vi>)  [unwired: 1 in]
        n213 = Unbundle By Name(w552) -> ("Event Registration Refnum"=w549:refnum<event-registration>)
        n214 = call "XY Graph Tipstrip Mouse Enter.vi"("Event Registration Refnum"=w549, "XY Graph Refnum"=w550) -> ("Event Registration Refnum"=w548:refnum<event-registration>)  [unwired: 8 in, 1 out]
        n215 = Bundle By Name(cluster=w552, "Event Registration Refnum"=w548) -> (w551:T3)
      }
      event Mouse Leave {
        n216 = event-data() -> ("CtlRef"=w555:refnum<vi>)  [unwired: 1 in]
        n217 = Unbundle By Name(w557) -> ("Event Registration Refnum"=w554:refnum<event-registration>)
        n218 = call "XY Graph Tipstrip Mouse Leave.vi"("Event Registration Refnum"=w554, "XY Graph Refnum"=w555) -> ("Event Registration Refnum"=w553:refnum<event-registration>)  [unwired: 8 in, 1 out]
        n219 = Bundle By Name(cluster=w557, "Event Registration Refnum"=w553) -> (w556:T3)
      }
      event Mouse Move {
        n220 = event-data() -> ("CtlRef"=w561:refnum<vi>, "Coords"=w560:T7)  [unwired: 1 in]
        n221 = call "XY Graph TipStrip Mouse Move.vi"("Coords"=w560, "XY Graph Refnum"=w561) -> ("Error Out"=w558:errorcluster)  [unwired: 7 in, 2 out]
        n222 = call <vilib>:"Clear Errors.vi"("error in (no error)"=w558) -> ()  [unwired: 5 in, 2 out]
      }
      event Menu Selection (User) {
        n223 = event-data() -> ("VIRef"=w567:refnum<vi>, "MenuRef"=w562:refnum<k9>, "ItemTag"=w566:string)  [unwired: 1 in]
        n224 = case shown="\"Close\"" w566 {
          tunnel: w567 -> [_ _ _ _ _ _ _ _ _ _]
          tunnel: w565 -> [_ w569 w572 _ _ _ _ _ _ _]
          tunnel: w564 -> [_ _ _ _ w573 w583 w591 w599 w607 w610]
          tunnel: [_ TRUE _ _ _ _ _ _ _ _] -> w563
          tunnel: w562 -> [_ _ _ _ w574 w580 w588 w593 w604 w608]
          frame "", Default {
          }
          frame "Close" {
            n225 = Enqueue Element(queue=w569, element=T1 {"Histogram Window Q Action"=enum."Quit", "Data"=variant} ("ALEX TT Histogram Q Element")) -> ()  [unwired: 2 in, 3 out]
          }
          frame "Export Graph to Notebook" {
            n226 = Enqueue Element(queue=w572, element=T1 {"Histogram Window Q Action"=enum."Export XYGraph to Notebook", "Data"=variant}) -> ()  [unwired: 2 in, 3 out]
          }
          frame "-------------" {
          }
          frame "Tool Panels" {
            n227 = call "XY Graph Show-Hide Tool Panels Event.vi"("XYGraph in"=w573) -> ("Error Out"=w575:errorcluster)  [unwired: 8 in, 2 out]
            n228 = call "Update Histogram Window Menu Checks.vi"("Error In"=w575, "menu reference"=w574, "XYGraph in"=w573) -> ()  [unwired: 8 in, 1 out]
          }
          frame "Plot Legend" {
            n229 = property class="XYGraph (strict)"(reference=w583) -> (reference out=w582:refnum<vi>, error out=w581:errorcluster, "Legend Visible"=w579:bool)  [unwired: 1 in]
            n230 = Not(x=w579) -> (.not. x?=w578:bool)
            n231 = property class="XYGraph (strict)"(reference=w582, error in=w581, "Legend Visible"=w578) -> (reference out=w577:refnum<vi>, error out=w576:errorcluster)
            n232 = call "Update Histogram Window Menu Checks.vi"("Error In"=w576, "menu reference"=w580, "XYGraph in"=w577) -> ()  [unwired: 8 in, 1 out]
          }
          frame "Graph Palette" {
            n233 = property class="XYGraph (strict)"(reference=w591) -> (reference out=w590:refnum<vi>, error out=w589:errorcluster, "Palette Visible"=w587:bool)  [unwired: 1 in]
            n234 = Not(x=w587) -> (.not. x?=w586:bool)
            n235 = property class="XYGraph (strict)"(reference=w590, error in=w589, "Palette Visible"=w586) -> (reference out=w585:refnum<vi>, error out=w584:errorcluster)
            n236 = call "Update Histogram Window Menu Checks.vi"("Error In"=w584, "menu reference"=w588, "XYGraph in"=w585) -> ()  [unwired: 8 in, 1 out]
          }
          frame "Scale Legend" {
            n237 = property class="XYGraph (strict)"(reference=w599) -> (reference out=w598:refnum<vi>, error out=w597:errorcluster, "ScaleLegendVis"=w596:bool)  [unwired: 1 in]
            n238 = Not(x=w596) -> (.not. x?=w595:bool)
            n239 = property class="XYGraph (strict)"(reference=w598, error in=w597, "ScaleLegendVis"=w595) -> (reference out=w594:refnum<vi>, error out=w592:errorcluster)
            n240 = call "Update Histogram Window Menu Checks.vi"("Error In"=w592, "menu reference"=w593, "XYGraph in"=w594) -> ()  [unwired: 8 in, 1 out]
          }
          frame "Cursor Legend" {
            n241 = property class="XYGraph (strict)"(reference=w607) -> (reference out=w606:refnum<vi>, error out=w605:errorcluster, "Cursor Palette Vis"=w603:bool)  [unwired: 1 in]
            n242 = Not(x=w603) -> (.not. x?=w602:bool)
            n243 = property class="XYGraph (strict)"(reference=w606, error in=w605, "Cursor Palette Vis"=w602) -> (reference out=w600:refnum<vi>, error out=w601:errorcluster)
            n244 = call "Update Histogram Window Menu Checks.vi"("Error In"=w601, "menu reference"=w604, "XYGraph in"=w600) -> ()  [unwired: 8 in, 1 out]
          }
          frame "Grid" {
            n245 = call "XY Graph Show-Hide Grid Event.vi"("XYGraph Ref in"=w610) -> ("Error Out"=w609:errorcluster)  [unwired: 7 in, 3 out]
            n246 = call "Update Histogram Window Menu Checks.vi"("Error In"=w609, "menu reference"=w608, "XYGraph in"=w610) -> ()  [unwired: 8 in, 1 out]
          }
        }
      }
      event Panel Close? {
        w613 = TRUE
        n247 = event-data() -> ()  [unwired: 1 in, 3 out]
        n248 = Enqueue Element(queue=w612, element=T1 {"Histogram Window Q Action"=enum."Quit", "Data"=variant} ("ALEX TT Histogram Q Element")) -> ()  [unwired: 2 in, 3 out]
        n249 = event-data("Discard?"=w613) -> ()  [unwired: 1 in, 1 out]
      }
    }
  }
  n250 = case shown="True" FALSE {
    frame False {
    }
    frame True {
      "Histogram Graph" <- cluster{"Axis":dbl[], "Histogram":dbl[]}[] [] ("Histogram Graph")
    }
  }
  n251 = Unregister For Events(event registration refnum=w5) -> ()  [unwired: 1 in, 1 out]
  n252 = invoke class="VI" method="FP.Close"(reference=w7) -> (reference out=w14:refnum<vi>, error out=w13:errorcluster)  [unwired: 2 in, 1 out]
  n253 = Close Reference(reference=w14, error in (no error)=w13) -> (error out=w4:errorcluster)
  n254 = call "Clear Error.vi"("Error In"=w4) -> ()  [unwired: 8 in, 1 out]
